vi "Remove Nodes by Filter.vi"(8 "error in (no error)":errorcluster, 10 "Filter class instructions":refnum<class "Filter.lvclass">, 11 "Tree Map Handle In":T1) -> (0 "error out":errorcluster, 3 "Tree Map Handle Out":T1)   [LabVIEW 2020, in "Blue Tree Map OpenSource.lvlib"]
doc: "Remove multiple nodes from a TreeMap using a user-provided filter.\n\n\n<B>Filter class instructions</B>\nThis is a user-provided class that provides instructions on how to filter nodes from the TreeMap.\nThe default parent class yields a no-op."
uses:
  Blue Tree Map OpenSource.lvlib
  Typedefs/Tree Map Handle.ctl
  Typedefs/Tree Map.ctl
  Typedefs/Tree Map Data.ctl
  Typedefs/Tree Node Data.ctl
  Typedefs/Attribute Map.ctl
  Classes/Filter/Filter.lvclass
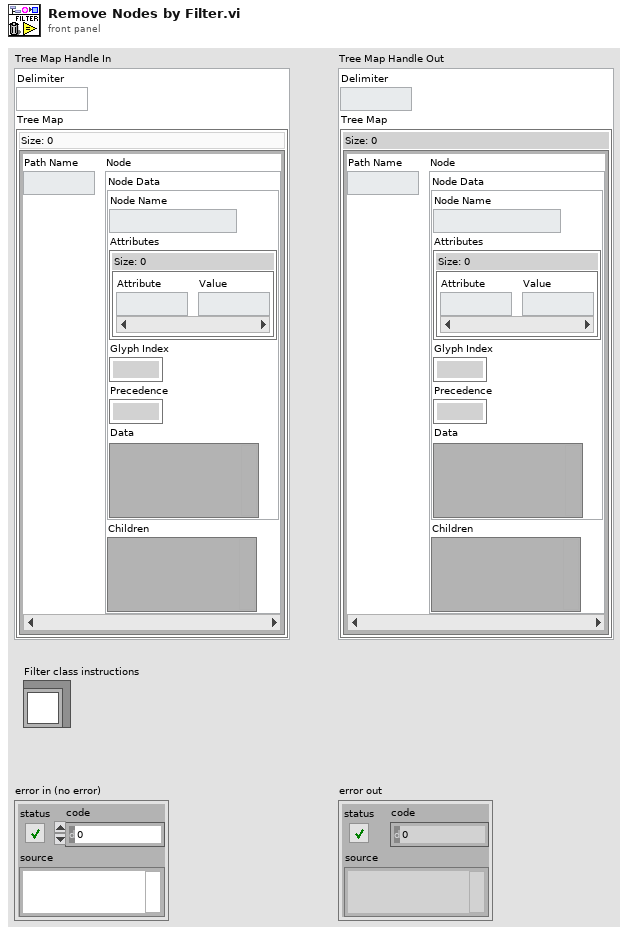
[diagram p1: front panel]
types:
  T1 = typedef "Blue Tree Map OpenSource.lvlib/Tree Map Handle.ctl" = cluster{"Delimiter":string, "Tree Map":T2}
  T2 = typedef "Blue Tree Map OpenSource.lvlib/Tree Map.ctl" = map{string, T3}
  T3 = typedef "Blue Tree Map OpenSource.lvlib/Tree Map Data.ctl" = cluster{"Node Data":T4, "Children":variant}
  T4 = typedef "Blue Tree Map OpenSource.lvlib/Tree Node Data.ctl" = cluster{"Node Name":string, "Attributes":T5, "Glyph Index":i32, "Precedence":i32, "Data":variant}
  T5 = typedef "Blue Tree Map OpenSource.lvlib/Attribute Map.ctl" = map{string, string}
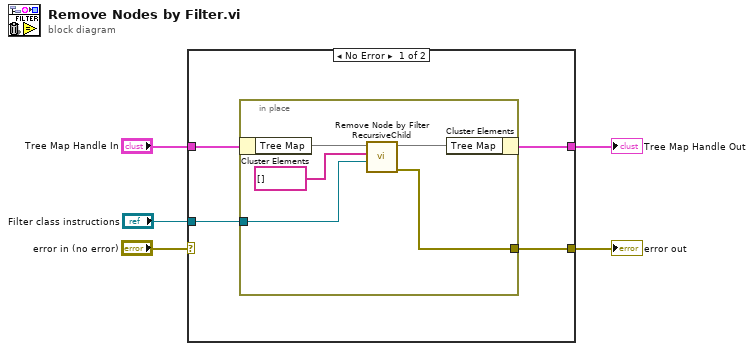
[diagram p0: block diagram]
diagram:
  n1 = case shown="No Error" "error in (no error)" {
    selector: "error in (no error)" -> [_ w16]
    tunnel: [w9 w16] -> w5
    tunnel: "Tree Map Handle In" -> [w8 w15]
    tunnel: [w7 w15] -> w3
    tunnel: "Filter class instructions" -> [w6 _]
    frame No Error {
      n2 = in-place {
        in-place-border: [w10] -> w9
        in-place-border: w6 -> [w11]
        n3 = in-place-cluster #1(w8) -> ("Tree Map"=w14:T2)
        n4 = call "Remove Node by Filter RecursiveChild.vi"("Filter class instructions"=w11, "Node Path (parent, child)"=string[] [], "Tree Map In"=w14) -> ("error out"=w10:errorcluster, "Tree Map Out"=w13:T2)  [unwired: 6 in, 1 out]
        n5 = in-place-cluster #1("Tree Map"=w13) -> (w7:T1)
      }
    }
    frame Error {
    }
  }
  "error out" <- w5
  "Tree Map Handle Out" <- w3
